vi "Error_Filter.vi"(8 "error in (no error)":errorcluster, 11 "Error Numbers To Filter":string) -> (0 "error out":errorcluster)   [LabVIEW 2015]
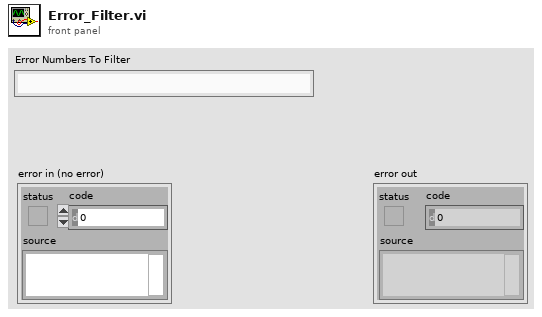
[diagram p1: front panel]
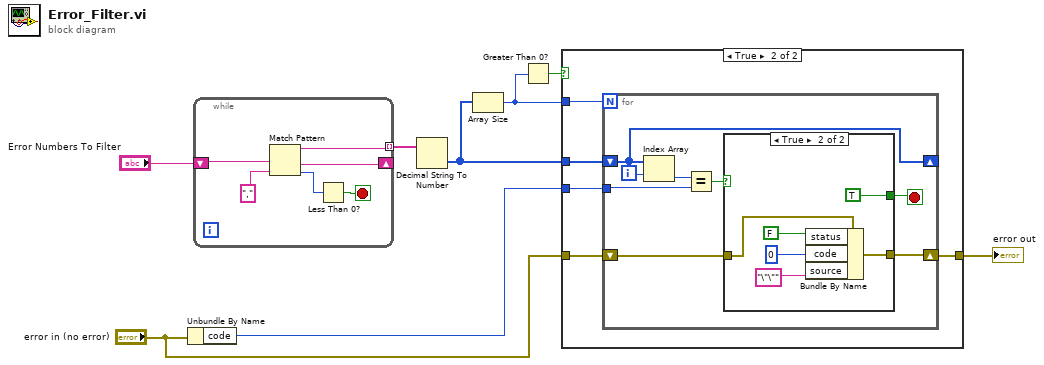
[diagram p0: block diagram]
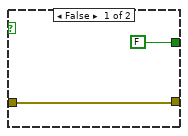
[diagram p3: hidden frame]
diagram:
  n1 = Unbundle By Name("error in (no error)") -> ("code"=w3:i32)
  n2 = while {
    tunnel: [w11] -> w8 mode=indexing
    shift-right: [w12] -> _
    shift-left: "Error Numbers To Filter" -> [w14]
    stop <- w9 stop-if-true
    n3 = Match Pattern(string=w14, regular expression=",") -> (before substring=w11:string, after substring=w12:string, offset past match=w10:i32)  [unwired: 2 out]
    n4 = Less Than 0?(x=w10) -> (x < 0?=w9:bool)
  }
  n5 = Decimal String To Number(string=w8) -> (number=w4:i32[])  [unwired: 3 out]
  n6 = Array Size(array=w4) -> (size(s)=w5:i32)
  n7 = Greater Than 0?(x=w5) -> (x > 0?=w6:bool)
  n8 = case shown="True" w6 {
    tunnel: w5 -> [_ w20]
    tunnel: w4 -> [_ w19]
    tunnel: w3 -> [_ w18]
    tunnel: "error in (no error)" -> [w15 w16]
    tunnel: [w15 w17] -> w1
    frame False {
    }
    frame True {
      n9 = for {
        N: w20 -> [_]
        tunnel: w18 -> [w26]
        shift-right: [w24] -> w17
        shift-left: w16 -> [w23]
        shift-right: [w21] -> _
        shift-left: w19 -> [w21]
        i -> [w28]
        stop <- w22 stop-if-true
        n10 = Index Array(array=w21, index=w28) -> (element=w27:i32)
        n11 = Equal?(x=w27, y=w26) -> (x = y?=w25:bool)
        n12 = case shown="True" w25 {
          tunnel: w23 -> [w30 w36]
          tunnel: [w30 w35] -> w24
          tunnel: [FALSE TRUE] -> w22
          frame False {
          }
          frame True {
            n13 = Bundle By Name(cluster=w36, "status"=FALSE, "code"=0, "source"="\"\"") -> (w35:errorcluster)
          }
        }
      }
    }
  }
  "error out" <- w1
